vi "Wait_for_capture.vi"(7 "error in (no error)":errorcluster, 10 "Initialize_card in":refnum<class "Control_card.lvclass">) -> (0 "error out":errorcluster, 2 "Progress":string, 3 "Initialize_card out":refnum<class "Control_card.lvclass">)   [LabVIEW 2015, in "Control_card.lvclass"]
uses:
  Control_card.lvclass
panel:
  in  "Abort":bool
  in  "Force Capture":bool
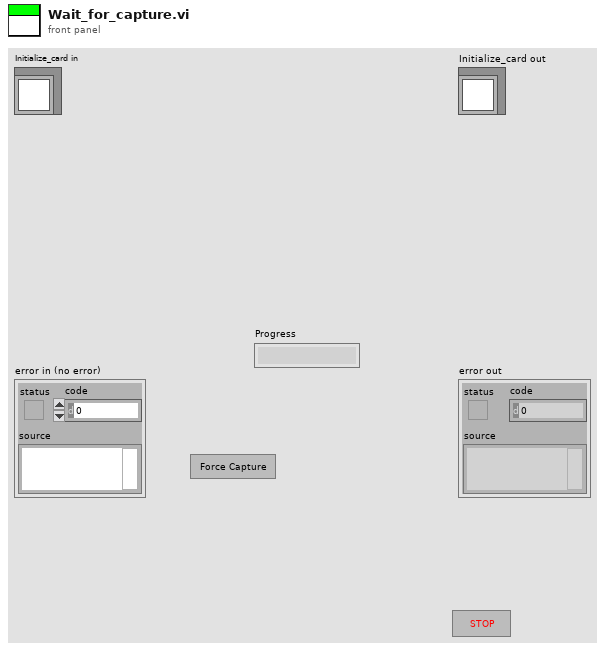
[diagram p1: front panel]
types:
  T1 = cluster{"Handle":u32, "Sample size":u32, "Resolution":i32, "Offset":i32, "Channels":u32, "Boards":u32}
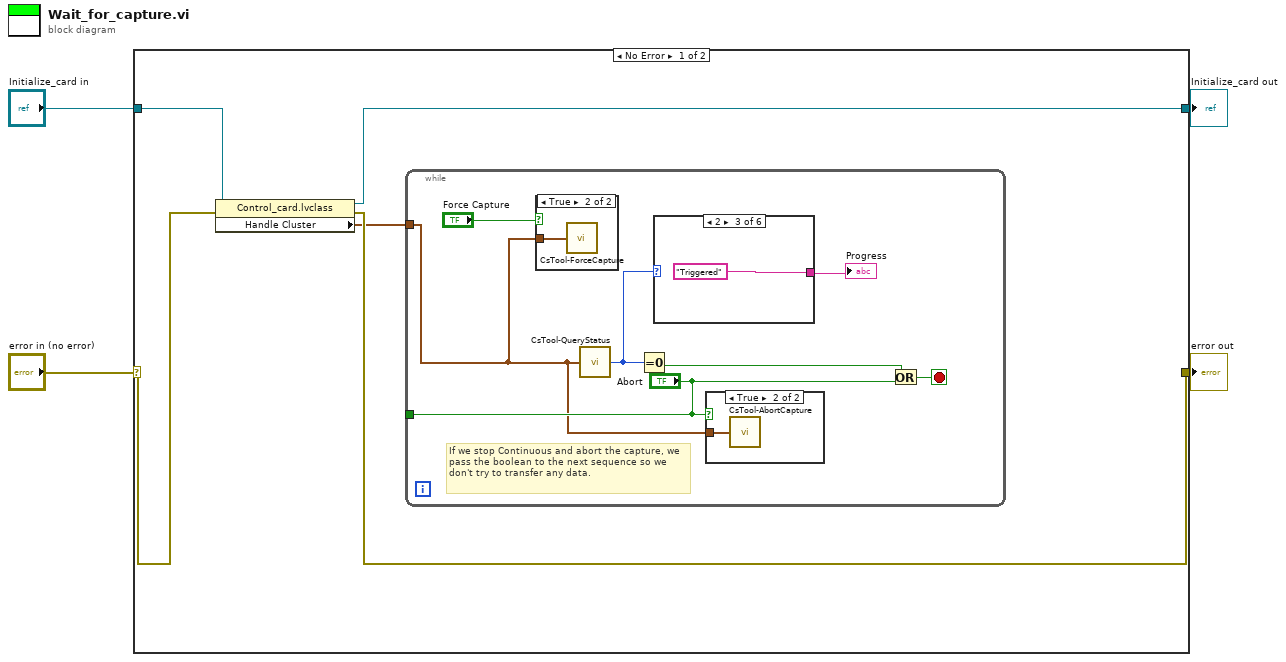
[diagram p0: block diagram]
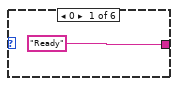
[diagram p4: hidden frame]
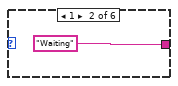
[diagram p5: hidden frame]
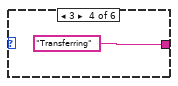
[diagram p6: hidden frame]
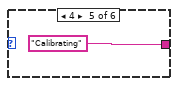
[diagram p7: hidden frame]
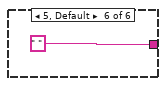
[diagram p8: hidden frame]
diagram:
  n1 = case shown="No Error" "error in (no error)" {
    selector: "error in (no error)" -> [w7 w26]
    tunnel: [w6 w26] -> w3
    tunnel: [w8 w25] -> w1
    tunnel: "Initialize_card in" -> [w9 w25]
    frame No Error {
      n2 = property class="Control_card.lvclass"(reference=w9, error in=w7) -> (reference out=w8:refnum<class "Control_card.lvclass">, error out=w6:errorcluster, "Handle Cluster"=w5:T1)
      n3 = while {
        tunnel: ["Abort"] -> _
        tunnel: w5 -> [w10]
        stop <- w13 stop-if-true
        # "If we stop Continuous and abort the capture, we pass the boolean to the next sequence so we don't try to transfer any data."
        n4 = case shown="True" "Force Capture" {
          tunnel: w10 -> [_ w17]
          frame False {
          }
          frame True {
            n5 = call <userlib>:"CsTool-ForceCapture.vi"("Handle Cluster"=w17) -> ()  [unwired: 1 out]
          }
        }
        n6 = call <userlib>:"CsTool-QueryStatus.vi"("Handle Cluster"=w10) -> ("Status"=w16:i32)
        n7 = Equal To 0?(x=w16) -> (x = 0?=w14:bool)
        n8 = case shown="2" w16 {
          tunnel: ["Ready" "Waiting" "Triggered" "Transferring" "Calibrating" " "] -> w15
          frame 0 {
          }
          frame 1 {
          }
          frame 2 {
          }
          frame 3 {
          }
          frame 4 {
          }
          frame 5, Default {
          }
        }
        "Progress" <- w15
        n9 = case shown="True" "Abort" {
          tunnel: w10 -> [_ w18]
          frame False {
          }
          frame True {
            n10 = call <userlib>:"CsTool-AbortCapture.vi"("Handle Cluster"=w18) -> ()  [unwired: 1 out]
          }
        }
        n11 = Or(x=w14, y="Abort") -> (x .or. y?=w13:bool)
      }
    }
    frame Error {
    }
  }
  "error out" <- w3
  "Initialize_card out" <- w1
